vi "Skyline Send Waveform File.vi"(8 "error in":errorcluster, 9 "properties":cluster{"Key":string, "Value":string}[](array[cluster]) caption="properties (null)", 11 "data in":waveform(dbl)[](array[waveform])) -> (0 "error out":errorcluster, 2 "size in bytes":i32, 3 "data out":waveform(dbl)[](array[waveform]))   [LabVIEW 2016]
uses:
  <vilib>/FileIngestion/Close (Single).vi
  <vilib>/FileIngestion/FileIngestion.lvlib
  <resource>/objmgr/FileIngestion.rc
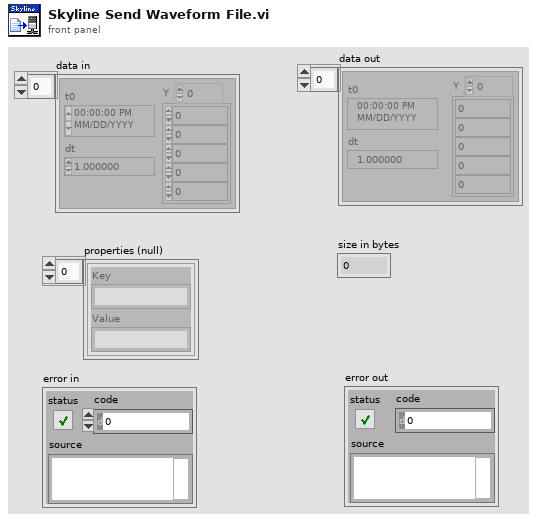
[diagram p1: front panel]
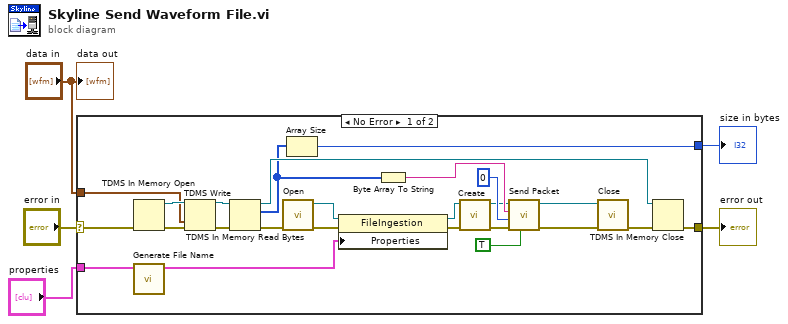
[diagram p0: block diagram]
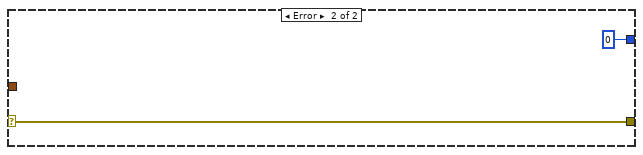
[diagram p2: hidden frame]
diagram:
  n1 = case shown="No Error" "error in" {
    selector: "error in" -> [w17 w32]
    tunnel: [w19 w32] -> w5
    tunnel: "properties" -> [w30 _]
    tunnel: "data in" -> [w28 _]
    tunnel: [w15 0] -> w1
    frame No Error {
      n2 = TDMS In Memory Open(8:w17) -> (0:w18:errorcluster, 3:w29:refnum<k34>)  [unwired: 1 in]
      n3 = call "Generate File Name.vi"("properties"=w30) -> ("Array"=w10:cluster{"Key":string, "Value":string}[])  [unwired: 10 in]
      n4 = TDMS Write(0:w29, 9:w28, 11:w18) -> (4:w26:refnum<k34>, 15:w27:errorcluster)  [unwired: 3 in, 2 out]
      n5 = TDMS In Memory Read Bytes(8:w27, 11:w26) -> (0:w23:errorcluster, 2:w16:u8[], 3:w25:refnum<k34>)  [unwired: 2 in]
      n6 = call <vilib>:"Open.vi"("error in"=w23) -> ("error out"=w11:errorcluster, "fileingestion refnum"=w12:refnum<k21>)  [unwired: 9 in]
      n7 = Array Size(array=w16) -> (size(s)=w15:i32)
      n8 = property class="FileIngestion"(reference=w12, error in=w11, "Properties"=w10) -> (reference out=w9:refnum<k21>, error out=w8:errorcluster)
      n9 = Byte Array To String(unsigned byte array=w16) -> (string=w24:string)
      n10 = call <vilib>:"Create.vi"("error in"=w8, "fileingestion refnum"=w9) -> ("error out"=w7:errorcluster, "fileingestion refnum out"=w6:refnum<k21>)  [unwired: 7 in]
      n11 = call <vilib>:"Send Packet.vi"("is last packet"=TRUE, "error in"=w7, "packet number"=0, "data"=w24, "fileingestion refnum in"=w6) -> ("error out"=w21:errorcluster, "fileingestion refnum out"=w22:refnum<k21>)  [unwired: 5 in]
      n12 = call-poly <vilib>:"Close.vi"("error in"=w21, "fileingestion refnum in"=w22) -> ("error out"=w20:errorcluster)  [unwired: 9 in]
      n13 = TDMS In Memory Close(8:w20, 11:w25) -> (0:w19:errorcluster)  [unwired: 2 in]
    }
    frame Error {
    }
  }
  "error out" <- w5
  "size in bytes" <- w1
  "data out" <- "data in"
